vi "nanomsg_geterr.vi"(1 "error in":errorcluster) -> (0 "type":T1)   [LabVIEW 2014, in "nanomsg.lvlib"]
doc: "Checks an error cluster for errors originating from Nanomsg, and returns an enum corresponding to which error it was."
uses:
  nanomsg.lvlib
  error_type.ctl
panel:
  # "NN"
  # "labview"
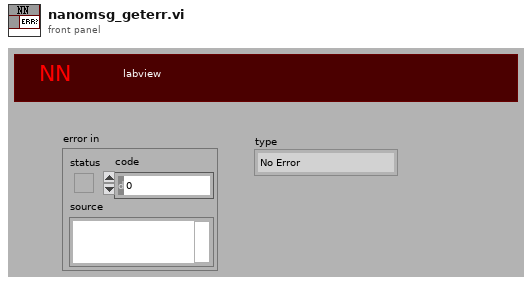
[diagram p1: front panel]
types:
  T1 = typedef "nanomsg.lvlib/error_type.ctl" = enum16{"No Error", "EUNKNOWN", "ENOTSUP", "EPROTONOSUPPORT", "ENOBUFS", "ENETDOWN", "EADDRINUSE", "EADDRNOTAVAIL", "ECONNREFUSED", "EINPROGRESS", "ENOTSOCK", "EAFNOSUPPORT", "EPROTO", "EAGAIN", "EBADF", "EINVAL", "EMFILE", "EFAULT", "EACCES", "ENETRESET", "ENETUNREACH", "EHOSTUNREACH", "ENOTCONN", "EMSGSIZE", "ETIMEDOUT", "ECONNABORTED", "ECONNRESET", "ENOPROTOOPT", "EISCONN", "ESOCKTNOSUPPORT", "EBUSY", "ENODEV", "EINTR", "ENOENT", "ENOMEM", "EFSM", "ETERM", "Invalid"}
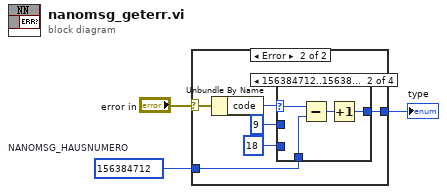
[diagram p0: block diagram]
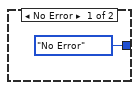
[diagram p2: hidden frame]
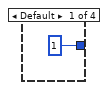
[diagram p3: hidden frame]
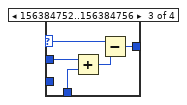
[diagram p4: hidden frame]
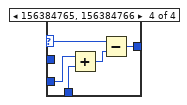
[diagram p5: hidden frame]
diagram:
  w1 = 156384712  # NANOMSG_HAUSNUMERO
  n1 = case shown="Error" "error in" {
    selector: "error in" -> [_ w9]
    tunnel: [error_type."No Error" ("type") w10] -> w3
    tunnel: w1 -> [_ w7]
    frame No Error {
    }
    frame Error {
      n2 = Unbundle By Name(w9) -> ("code"=w8:i32)
      n3 = case shown="156384712..156384740" w8 {
        selector: w8 -> [_ w15 w19 w24]
        tunnel: [1 w12 w20 w23] -> w10
        tunnel: w7 -> [_ w13 w17 w22]
        tunnel: 9 ("x") -> [_ _ w16 _]
        tunnel: 18 ("x") -> [_ _ _ w21]
        frame Default {
        }
        frame 156384712..156384740 {
          n4 = Subtract(x=w15, y=w13) -> (x-y=w14:i32)
          n5 = Increment(x=w14) -> (x+1=w12:i32)
        }
        frame 156384752..156384756 {
          n6 = Add(x=w16, y=w17) -> (x+y=w18:i32)
          n7 = Subtract(x=w19, y=w18) -> (x-y=w20:i32)
        }
        frame 156384765, 156384766 {
          n8 = Add(x=w21, y=w22) -> (x+y=w25:i32)
          n9 = Subtract(x=w24, y=w25) -> (x-y=w23:i32)
        }
      }
    }
  }
  "type" <- w3
